vi "RDV-addDataToMap.vi"(7 "Folder Path":path=path "C:/projects/Universitet/Master/data/Real Test - First libreVNA test with calibration file/Converted Data", 8 "error in (no error)":errorcluster, 11 "RDV-Reflection_Data_viewer in":refnum<class "RDV-Reflection_Data_viewer.lvclass">) -> (0 "error out":errorcluster, 3 "RDV-Reflection_Data_viewer out":refnum<class "RDV-Reflection_Data_viewer.lvclass">)   [LabVIEW 2020, in "RDV-Reflection_Data_viewer.lvclass"]
uses:
  RDV-Reflection_Data_viewer.lvclass
  RDV-Reflection_Data_viewer.lvclass/RDV-Reflection_Data_viewer.ctl
  Tools/Reflector/RFH-Reflection_File_Handler.lvlib
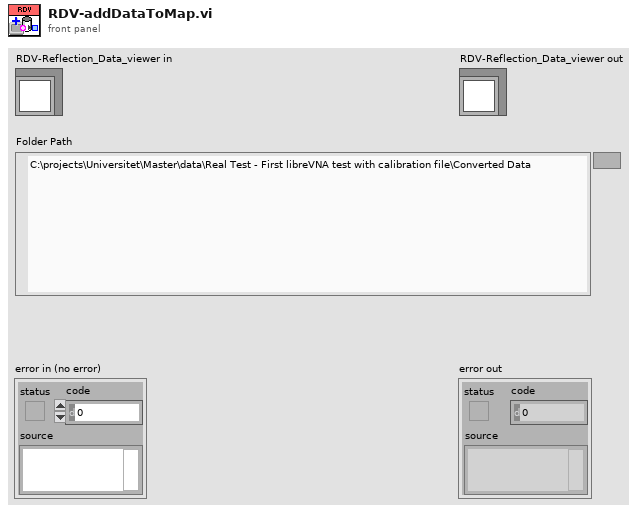
[diagram p1: front panel]
types:
  T1 = typedef "RDV-Reflection_Data_viewer.lvclass/RDV-DATA_MAP.ctl" = map{string, cluster{"filename without extension":string, "Common Format":T2}}
  T2 = typedef "RFH-Reflection_File_Handler.lvlib/RFH-common_data_format.ctl" = cluster{"Frequency":dbl[], "Reflection'":dbl[], "Reflection''":dbl[], "Permativity'":dbl[], "Permativity''":dbl[]}
  T3 = cluster{"filename without extension":string, "Common Format":T2}
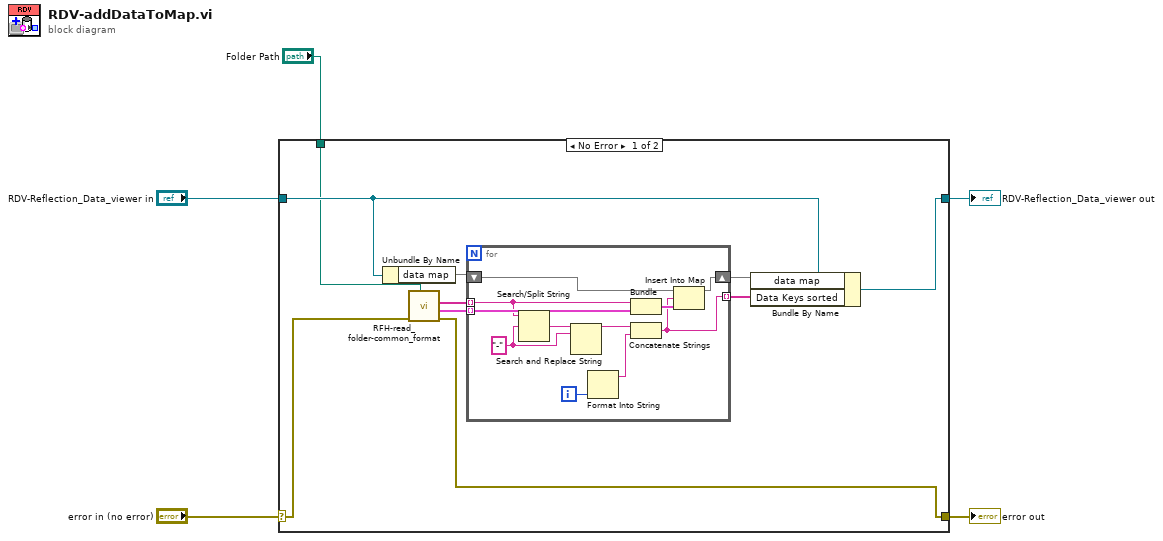
[diagram p0: block diagram]
diagram:
  n1 = case shown="No Error" "error in (no error)" {
    selector: "error in (no error)" -> [w6 w28]
    tunnel: [w7 w28] -> w4
    tunnel: [w9 w27] -> w2
    tunnel: "RDV-Reflection_Data_viewer in" -> [w10 w27]
    tunnel: "Folder Path" -> [w8 _]
    frame No Error {
      n2 = Unbundle By Name(w10) -> ("data map"=w13:T1)
      n3 = call "RFH-read_folder-common_format.vi"("Folder Path"=w8, "error In"=w6) -> ("error out"=w7:errorcluster, "Data"=w14:T2[], "Names"=w15:string[])  [unwired: 7 in]
      n4 = for {
        tunnel: w15 -> [w17] mode=indexing
        tunnel: [w16] -> w11 mode=indexing
        tunnel: w14 -> [w24] mode=indexing
        shift-right: [w21] -> w12
        shift-left: w13 -> [w23]
        i -> [w20]
        w25 = "-" ("search string/char (-)")
        n5 = Search/Split String(string=w17, search string/char (-)=w25) -> (match + rest of string=w26:string)  [unwired: 1 in, 2 out]
        n6 = Search and Replace String(input string=w26, search string=w25) -> (result string=w19:string)  [unwired: 6 in, 3 out]
        n7 = Format Into String(w20) -> (resulting string=w18:string)  [unwired: 3 in, 1 out]
        n8 = Bundle("filename without extension"=w17, "Common Format"=w24) -> (w22:T3)  [unwired: 1 in]
        n9 = Concatenate Strings(w19, w18) -> (w16:string)
        n10 = Insert Into Map(map in=w23, key=w16, value=w22) -> (map out=w21:T1)  [unwired: 2 out]
      }
      n11 = Bundle By Name(cluster=w10, "data map"=w12, "Data Keys sorted"=w11) -> (w9:refnum<class "RDV-Reflection_Data_viewer.lvclass">)
    }
    frame Error {
    }
  }
  "error out" <- w4
  "RDV-Reflection_Data_viewer out" <- w2
